vi "initializeArrayElement.vi"(8 "error in (no error)":errorcluster, 9 "arraySize":u16, 10 "arrayRef":refnum<vi>, 11 "Numeric in":refnum<class "Numeric.lvclass">) -> (0 "error out":errorcluster, 3 "Numeric out":refnum<class "Numeric.lvclass">)   [LabVIEW 2016, in "Numeric.lvclass"]
uses:
  Numeric.lvclass
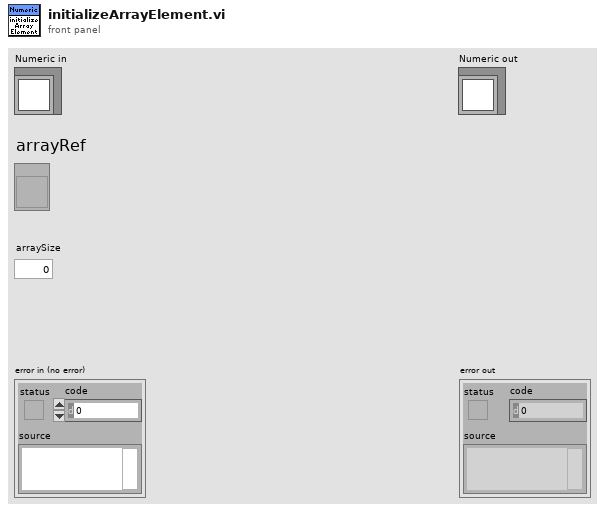
[diagram p1: front panel]
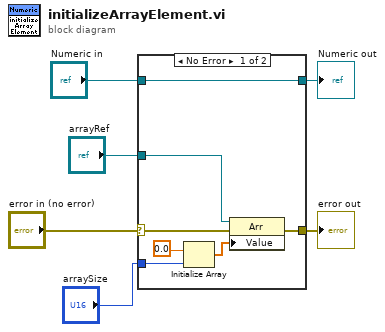
[diagram p0: block diagram]
diagram:
  n1 = case shown="No Error" "error in (no error)" {
    selector: "error in (no error)" -> [w11 w15]
    tunnel: [w10 w15] -> w5
    tunnel: "arraySize" -> [w9 _]
    tunnel: [w8 w14] -> w3
    tunnel: "Numeric in" -> [w8 w14]
    tunnel: "arrayRef" -> [w7 _]
    frame No Error {
      n2 = Initialize Array(0.0 ("element"), w9) -> (w12:dbl[])
      n3 = property class="Arr"(reference=w7, error in=w11, "Value"=w12) -> (error out=w10:errorcluster)  [unwired: 1 out]
    }
    frame Error {
    }
  }
  "error out" <- w5
  "Numeric out" <- w3
